vi "SSC DCPower Get Max Current.vi"(0 "DCPower SSC in":T1[](array[typedef]), 11 "error in":errorcluster) -> (4 "DCPower SSC out":T1[](array[typedef]), 6 "Max Current":dbl[](array[numeric]) format="%#_6p", 15 "error out":errorcluster)   [LabVIEW 2019]
doc: "This VI returns the max Current (A) Range for each DCPower Session."
uses:
  SSC DCPower.ctl
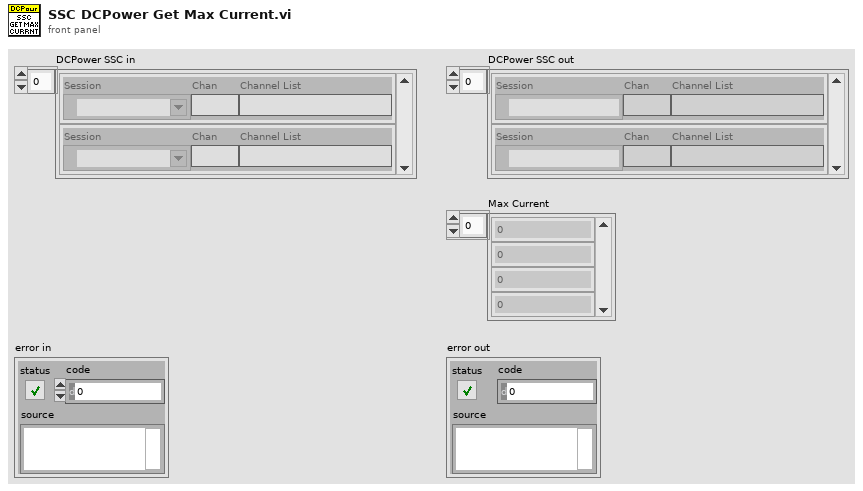
[diagram p1: front panel]
types:
  T1 = typedef "SSC DCPower.ctl" = cluster{"Session":refnum<k15>, "Chan":string, "Channel List":string}
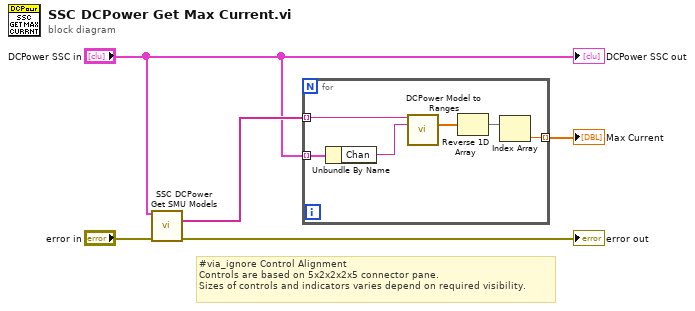
[diagram p0: block diagram]
diagram:
  # "#via_ignore Control Alignment\nControls are based on 5x2x2x2x5 connector pane.\nSizes of controls and indicators varies depend on required visibility."
  n1 = call "SSC DCPower Get SMU Models.vi"("DCPower SSC in"="DCPower SSC in", "error in"="error in") -> ("SMU Models"=w4:string[], "error out"=→"error out":errorcluster)  [unwired: 11 in, 1 out]
  n2 = for {
    tunnel: w4 -> [w11] mode=indexing
    tunnel: [w8] -> w2 mode=indexing
    tunnel: "DCPower SSC in" -> [w7] mode=indexing
    n3 = Unbundle By Name(w7) -> ("Chan"=w6:string)
    n4 = call "DCPower Model to Ranges.vi"("SMU Model"=w11, "Channel"=w6) -> ("Current Ranges (A)"=w10:dbl[])  [unwired: 11 in, 2 out]
    n5 = Reverse 1D Array(array=w10) -> (reversed array=w9:dbl[])
    n6 = Index Array(array=w9) -> (element=w8:dbl)  [unwired: 1 in]
  }
  "Max Current" <- w2
  "DCPower SSC out" <- "DCPower SSC in"
